vi "Phi from quaternions (SubVI).vi"(6 "Array in":dbl[](array[numeric]), 9 "Array 3":dbl[](array[numeric]), 10 "Array 4":dbl[](array[numeric]), 11 "Array 5":dbl[](array[numeric])) -> (3 "Array out":dbl[](array[numeric]))   [LabVIEW 2011]
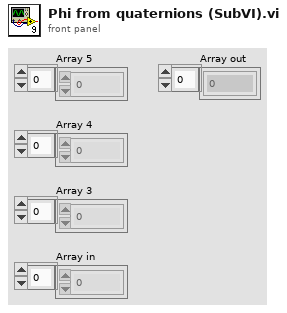
[diagram p1: front panel]
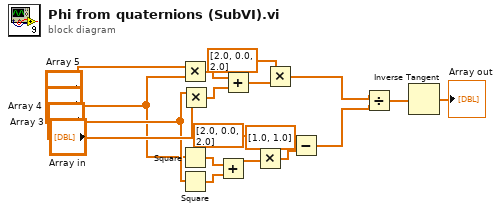
[diagram p0: block diagram]
diagram:
  n1 = Multiply(x="Array 5", y="Array 4") -> (x*y=w6:dbl[])
  n2 = Square(x="Array 4") -> (x^2=w1:dbl[])
  n3 = Square(x="Array 3") -> (x^2=w2:dbl[])
  n4 = Multiply(x="Array 3", y="Array in") -> (x*y=w5:dbl[])
  n5 = Add(x=w1, y=w2) -> (x+y=w3:dbl[])
  n6 = Add(x=w6, y=w5) -> (x+y=w4:dbl[])
  n7 = Multiply(x=dbl[] [2.0, 0.0, 2.0], y=w3) -> (x*y=w7:dbl[])
  n8 = Multiply(x=dbl[] [2.0, 0.0, 2.0], y=w4) -> (x*y=w8:dbl[])
  n9 = Subtract(x=dbl[] [1.0, 1.0], y=w7) -> (x-y=w9:dbl[])
  n10 = Divide(x=w8, y=w9) -> (x/y=w17:dbl[])
  n11 = Inverse Tangent(1:w17) -> (0:→"Array out":dbl[])
